vi "Button Press Listener.vi"(8 "error in (no error)":errorcluster, 10 "I/O Data":refnum<user-event>, 11 "DaqMX task":refnum<k21>) -> ()   [LabVIEW 2025]
uses:
  <vilib>/DAQmx/read.llb/DAQmx Read (Digital 1D Bool NChan 1Samp 1Line).vi
  <vilib>/DAQmx/miscellaneous.llb/DAQmx Fill In Error Info.vi
panel:
  out "n":i32 caption="#Events Fired"
  out "Button States":bool[](array[boolean])
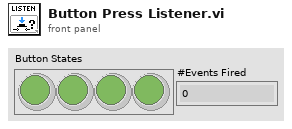
[diagram p1: front panel]
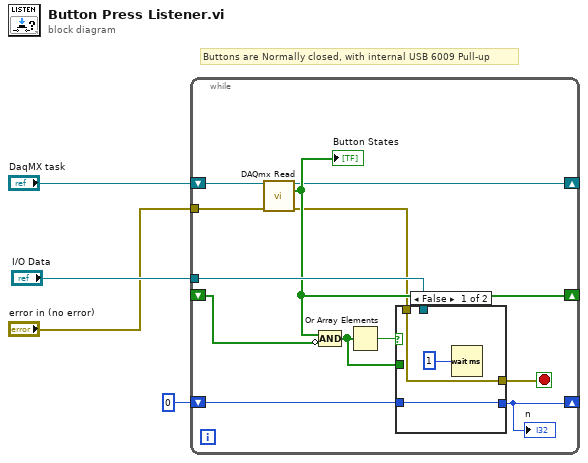
[diagram p0: block diagram]
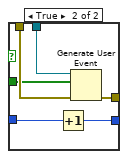
[diagram p2: hidden frame]
diagram:
  # "Buttons are Normally closed, with internal USB 6009 Pull-up"
  n1 = while {
    tunnel: "error in (no error)" -> [w15]
    tunnel: "I/O Data" -> [w13]
    shift-right: [w12] -> _
    shift-left: _ -> [w14]
    shift-right: [w8] -> _
    shift-left: "DaqMX task" -> [w16]
    shift-right: [w6] -> _
    shift-left: 0 -> [w5]
    stop <- w11 stop-if-true
    n2 = call-poly <vilib>:"DAQmx Read.vi"("task/channels in"=w16, "error in"=w15) -> ("task out"=w8:refnum<k21>, "data"=w12:bool[], "error out"=w10:errorcluster)  [unwired: 11 in]
    "Button States" <- w12
    n3 = Compound Arithmetic op=AND(w12, invert w14) -> (w7:bool[])
    n4 = Or Array Elements(Boolean array=w7) -> (logical OR=w9:bool)
    n5 = case shown="False" w9 {
      tunnel: w13 -> [_ w25]
      tunnel: [w19 w24] -> w11
      tunnel: w10 -> [w19 w23]
      tunnel: w7 -> [_ w22]
      tunnel: [w17 w21] -> w6
      tunnel: w5 -> [w17 w20]
      frame False {
        n6 = Wait (ms)(milliseconds to wait=u32 1) -> ()  [unwired: 1 out]
      }
      frame True {
        n7 = Increment(x=w20) -> (x+1=w21:i32)
        n8 = Generate User Event(user event=w25, event data cluster=w22, error in=w23) -> (error out=w24:errorcluster)  [unwired: 1 in, 1 out]
      }
    }
    "n" <- w6
  }
